vi "Send Configure Trigger Slope [TS].vi"(7 "Message Priority (Normal)":T1=enum."Normal", 8 "error in (no error)":errorcluster, 10 "trigger slope (0: Positive)":i32(ring) items=["Positive", "Negative"], 11 "Message Enqueuer":refnum<class "Message Enqueuer.lvclass">) -> (0 "error out":errorcluster, 3 "Message Enqueuer out":refnum<class "Message Enqueuer.lvclass">)   [LabVIEW 2015, in "CS++DMM.lvlib" / "Configure Trigger Slope [TS] Msg.lvclass"]
doc: "Sends the <B>CS++DMM.lvlib:Configure Trigger Slope [TS] Msg.lvclass</B> message.\n\n<B>CS++DMM.lvlib:CS++DMM.lvclass:Configure Trigger Slope [TS].vi</B> Description:\n\nThis VI configures the polarity of the external trigger source of the DMM.\n\nNote:\n\n(1) This VI is part of the IviDmmTriggerSlope [TS] extension group."
uses:
  Configure Trigger Slope [TS] Msg.lvclass
  <vilib>/ActorFramework/Message Enqueuer/Message Enqueuer.lvclass
  <vilib>/ActorFramework/Message Enqueuer/Message Priority.ctl
  Configure Trigger Slope [TS] Msg.lvclass/Configure Trigger Slope [TS] Msg.ctl
  <vilib>/ActorFramework/Message Enqueuer/Message Enqueuer.lvclass/Message Enqueuer.ctl
  <vilib>/ActorFramework/Message Priority Queue/Priority Enqueue.vi
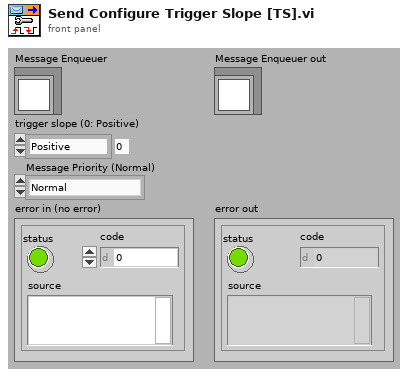
[diagram p1: front panel]
types:
  T1 = typedef "Actor Framework.lvlib/Message Enqueuer.lvclass/Message Priority.ctl" = enum16{"Low", "Normal", "High"}
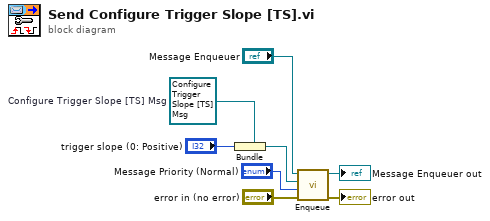
[diagram p0: block diagram]
diagram:
  w2 = refnum<class "Configure Trigger Slope [TS] Msg.lvclass"> refnum  # Configure Trigger Slope [TS] Msg
  n1 = Bundle(cluster=w2, "trigger slope (0: Positive)") -> (w5:refnum<class "Configure Trigger Slope [TS] Msg.lvclass">)
  n2 = call <vilib>:"Enqueue.vi"("error in (no error)"="error in (no error)", "Message Priority (Normal)"="Message Priority (Normal)", "Message"=w5, "Message Enqueuer in"="Message Enqueuer") -> ("error out"=→"error out":errorcluster, "Message Enqueuer out"=→"Message Enqueuer out":refnum<class "Message Enqueuer.lvclass">)  [unwired: 6 in]
